vi "ModeMgr.Setup Utility.vi"() -> ()   [LabVIEW 2018]
uses:
  ModeMgr.Mode Settings.ctl
  ModeMgr.ModeConfig.ctl
  ModeMgr.Mode Settings_Config View.ctl
panel:
  in  "Delete Mode":bool
  in  "Mode List":i32(listbox)
  out "Option Descriptions":cluster{"Option":string, "Desc":string}[](array[cluster])=[{"Option"="Can Access Station Module", "Desc"="Level 0 = the button and menu item to open the station control module is not available.  Level 1 (or higher) = the station module can be opened."}, {"Option"="Can Clear Errors", "Desc"="Level 0 = the button to clear errors is disabled.  Level 1 (or higher) = the button to clear errors is enabled."}, {"Option"="Can Clear Warnings", "Desc"="Level 0 = the button to clear warnings is disabled.  Level 1 (or higher) = the button to clear warnings is enabled."}, {"Option"="Can Edit EQ List", "Desc"="Level 0 = the Equipment list can not be edited.  Level 1 (or higher) = the Equipment list can be edited."}, {"Option"="Can Edit Options", "Desc"="Level 0 = the controls for options (on tab page Config - Options) is disabled.  Level 1 (or higher) = the controls for options (on tab page Config - Options) is enabled."}, {"Option"="Can Generate Reports", "Desc"="Level 0 = the controls to generate RTF or CSV reports are disabled.  Level 1 (or higher) = the controls to generate RTF or CSV reports are enabled."}, {"Option"="Can Select Sequence", "Desc"="Level 0 = the controls for selecting the test sequence is disabled.  The default sequence (configured) is the only available sequenct that can be run. Level 1 (or higher) = the sequence selector control is enabled."}, {"Option"="Can View Config", "Desc"="Level 0 = the tab page for Config is hidden.  Level 1 (or higher) = the tab page for Config is visible and can eb selected."}, {"Option"="Disable Results", "Desc"="Level 0 = test results are reported for each test 9to Factory and to Data Warehouse).  Level 1 (or higher) = no results are reported."}, {"Option"="Disable Start with SN Entry", "Desc"="Level 0 = the control to auto start test when a SN is entered is set to ON and can not be changed.  Level 1 (or higher) = the control to auto start test when a SN is entered is set to OFF and can be changed by the operator."}, {"Option"="Display Result Data Details", "Desc"="\"Level 0 =  The operator can only view the summary page.  Level 1 (or higher) = the tabs of the result section will be displayed and the operator can select to view the Summary"}, {"Option"="Not Reset SN between Tests", "Desc"="Level 0 = the SN field is cleared between tests.  Level 1 (or higher) = the SN remains the same between tests."}, {"Option"="Not Validate Operator", "Desc"="Level 0 = the operator field can not be empty.  The Start button is disabled until the operator field is populated.  Level 1 (or higher) = the operator can be empty."}, {"Option"="Not Validate SN", "Desc"="Level 0 = the SN field can not be empty.  The Start button is disabled until the SN field is populated.  Level 1 (or higher) = the SN can be empty."}]
  in  "Add Mode":bool
  out "Options":string[](array[string])=["Option", "Display Result Data Details", "Not Reset SN between Tests", "Not Validate Operator", "Not Validate SN", "Disable Results", "Can Access Station Module", "Can Edit EQ List", "Can Clear Warnings", "Can Clear Errors", "Can View Config", "Can Edit Options", "Can Select Sequence", "Can Generate Reports", "Disable Start with SN Entry"]
  out "Options File":path
  out "Ver":string
  in  "Save":bool
  in  "Load":bool
  in  "Mode Config":cluster{"Default Mode":string, "Modes":T1[]}={"Default Mode"="Production", "Modes"=[{"Name"="Production", "Color"=3, "Options"=[{"Option"="Can Access Station Module", "Level"=0}, {"Option"="Can Clear Errors", "Level"=0}, {"Option"="Can Clear Warnings", "Level"=0}, {"Option"="Can Edit EQ List", "Level"=0}, {"Option"="Can Edit Options", "Level"=0}, {"Option"="Can Generate Reports", "Level"=0}, {"Option"="Can Select Sequence", "Level"=0}, {"Option"="Can View Config", "Level"=0}, {"Option"="Disable Results", "Level"=0}, {"Option"="Disable Start with SN Entry", "Level"=0}, {"Option"="Display Result Data Details", "Level"=0}, {"Option"="Not Reset SN between Tests", "Level"=0}, {"Option"="Not Validate Operator", "Level"=0}, {"Option"="Not Validate SN", "Level"=0}], "Password"=""}, {"Name"="Technician", "Color"=1, "Options"=[{"Option"="Can Access Station Module", "Level"=0}, {"Option"="Can Clear Errors", "Level"=1}, {"Option"="Can Clear Warnings", "Level"=1}, {"Option"="Can Edit EQ List", "Level"=0}, {"Option"="Can Edit Options", "Level"=0}, {"Option"="Can Generate Reports", "Level"=1}, {"Option"="Can Select Sequence", "Level"=1}, {"Option"="Can View Config", "Level"=0}, {"Option"="Disable Results", "Level"=0}, {"Option"="Disable Start with SN Entry", "Level"=1}, {"Option"="Display Result Data Details", "Level"=1}, {"Option"="Not Reset SN between Tests", "Level"=1}, {"Option"="Not Validate Operator", "Level"=1}, {"Option"="Not Validate SN", "Level"=0}], "Password"=""}, {"Name"="Gage R&R", "Color"=6, "Options"=[{"Option"="Can Access Station Module", "Level"=0}, {"Option"="Can Clear Errors", "Level"=0}, {"Option"="Can Clear Warnings", "Level"=0}, {"Option"="Can Edit EQ List", "Level"=0}, {"Option"="Can Edit Options", "Level"=0}, {"Option"="Can Generate Reports", "Level"=0}, {"Option"="Can Select Sequence", "Level"=0}, {"Option"="Can View Config", "Level"=0}, {"Option"="Disable Results", "Level"=0}, {"Option"="Disable Start with SN Entry", "Level"=0}, {"Option"="Display Result Data Details", "Level"=0}, {"Option"="Not Reset SN between Tests", "Level"=0}, {"Option"="Not Validate Operator", "Level"=0}, {"Option"="Not Validate SN", "Level"=0}], "Password"=""}, {"Name"="Engineering", "Color"=4, "Options"=[{"Option"="Can Access Station Module", "Level"=1}, {"Option"="Can Clear Errors", "Level"=1}, {"Option"="Can Clear Warnings", "Level"=1}, {"Option"="Can Edit EQ List", "Level"=1}, {"Option"="Can Edit Options", "Level"=1}, {"Option"="Can Generate Reports", "Level"=1}, {"Option"="Can Select Sequence", "Level"=1}, {"Option"="Can View Config", "Level"=1}, {"Option"="Disable Results", "Level"=1}, {"Option"="Disable Start with SN Entry", "Level"=1}, {"Option"="Display Result Data Details", "Level"=1}, {"Option"="Not Reset SN between Tests", "Level"=1}, {"Option"="Not Validate Operator", "Level"=1}, {"Option"="Not Validate SN", "Level"=1}], "Password"=""}]} {"Modes"."Color" items=["Red", "Yellow", "Orange", "Green", "SkyBlue", "Blue", "Purple", "Pink", "Grey"]}
  # "MTE Mode Setup Utility"
  # "Option                                                                                             Description"
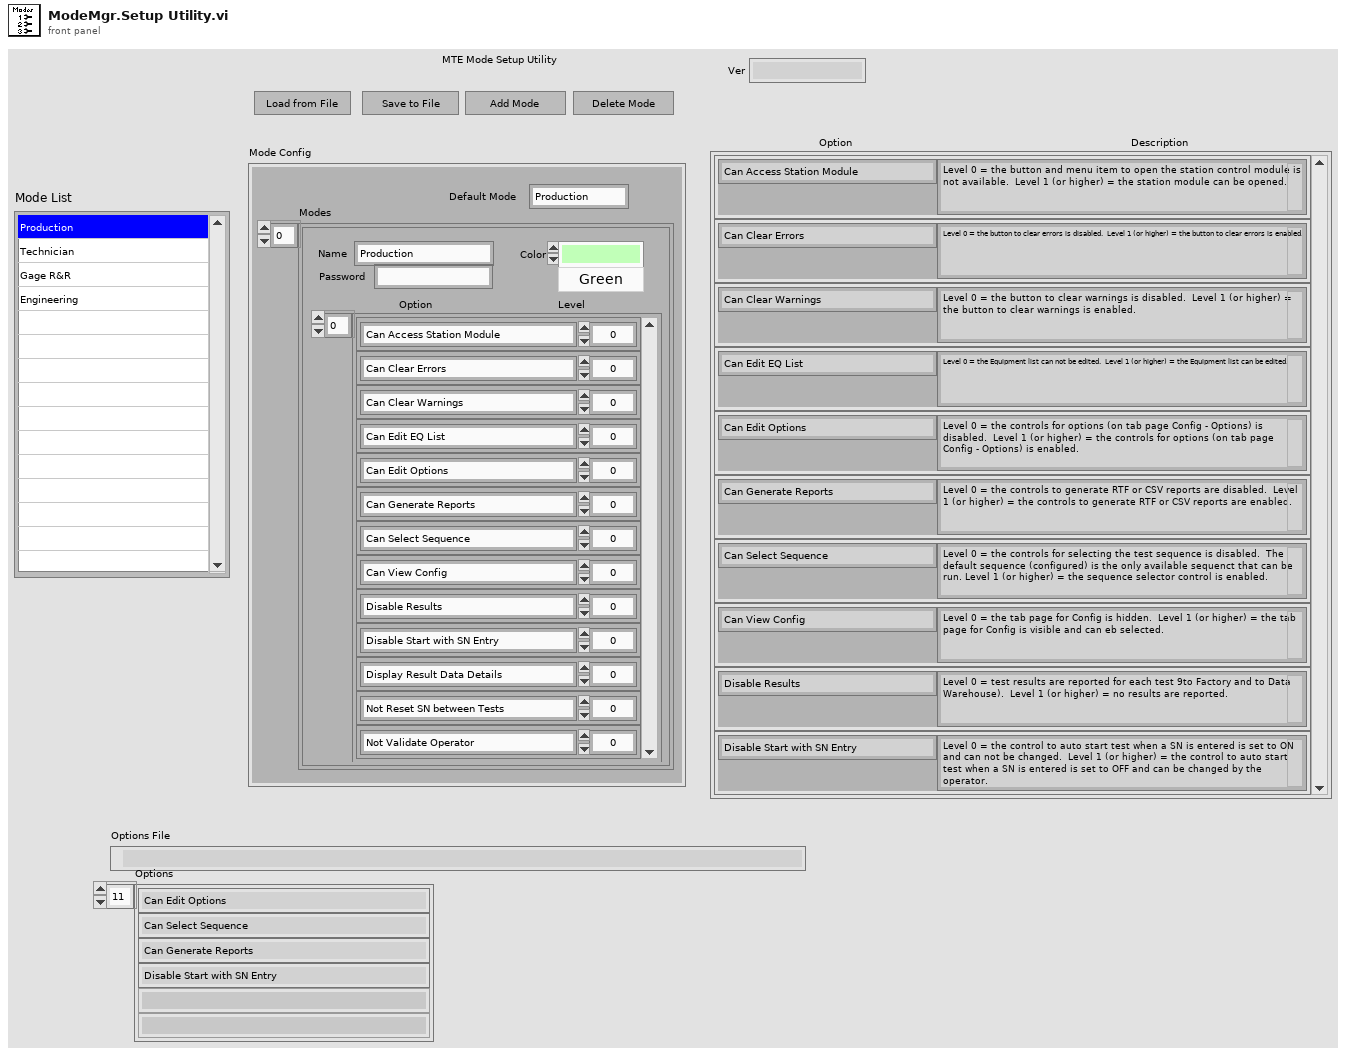
[diagram p1: front panel]
types:
  T1 = typedef "ModeMgr.Mode Settings_Config View.ctl" = cluster{"Name":string, "Color":u16, "Options":T2[], "Password":string}
  T2 = typedef "ModeMgr.Mode Settings.ctl" = cluster{"Option":string, "Level":i32}
  T3 = enum32{"invalid app kind", "Development System", "Run Time System", "Student Edition", "Embedded LabVIEW", "Evaluation", "Custom"}
  T4 = typedef "ModeMgr.ModeConfig.ctl" = cluster{"Name":string, "Color":string, "Settings":T2[], "Password":string}
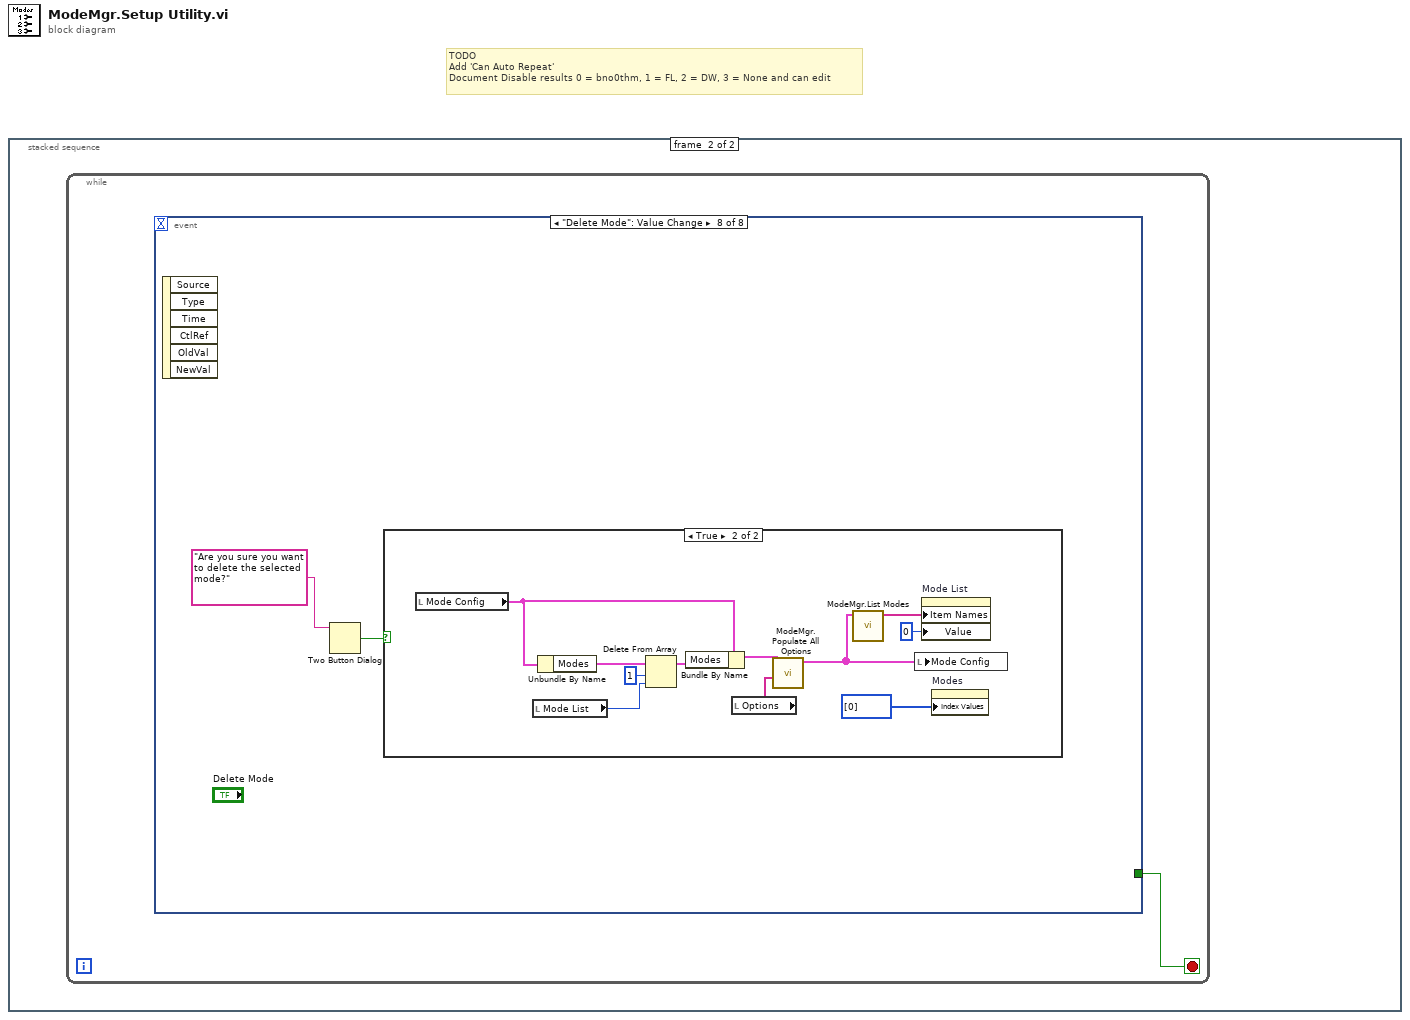
[diagram p0: block diagram]
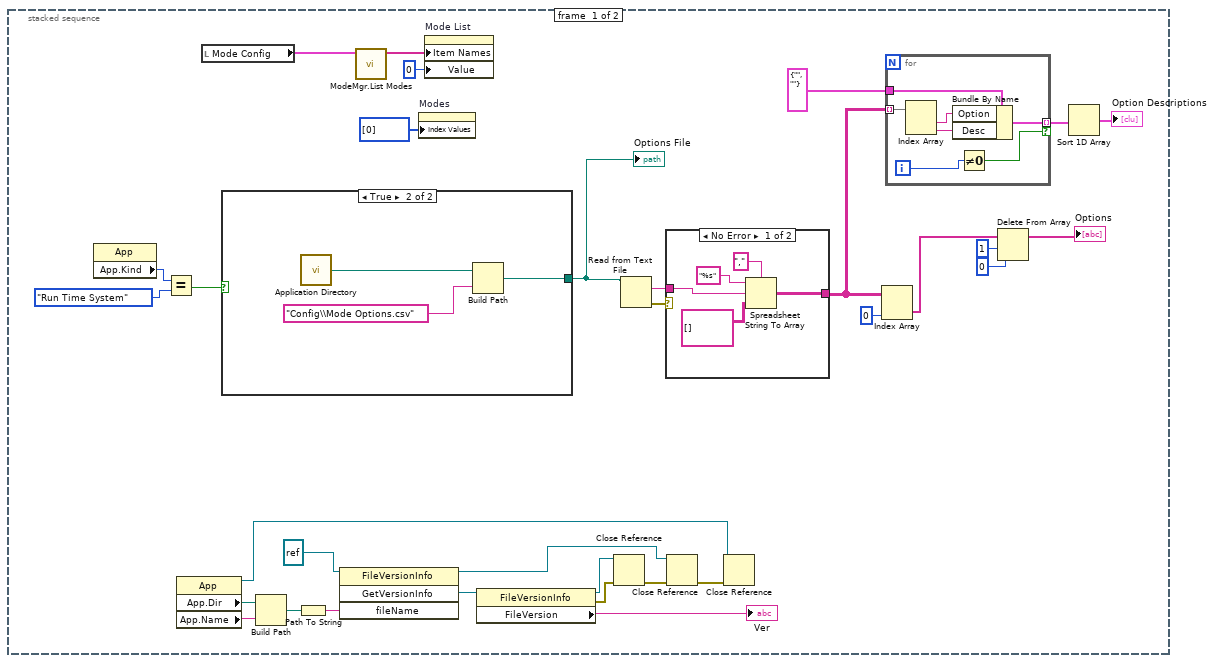
[diagram p2: hidden frame]
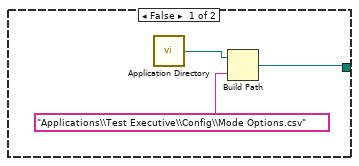
[diagram p4: hidden frame]
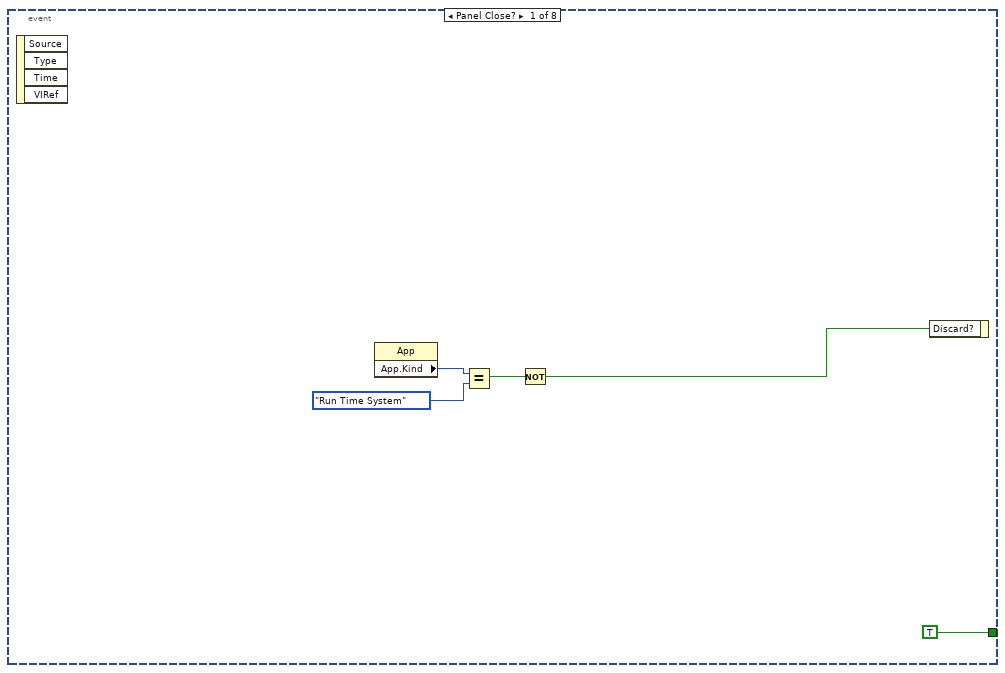
[diagram p5: hidden frame]
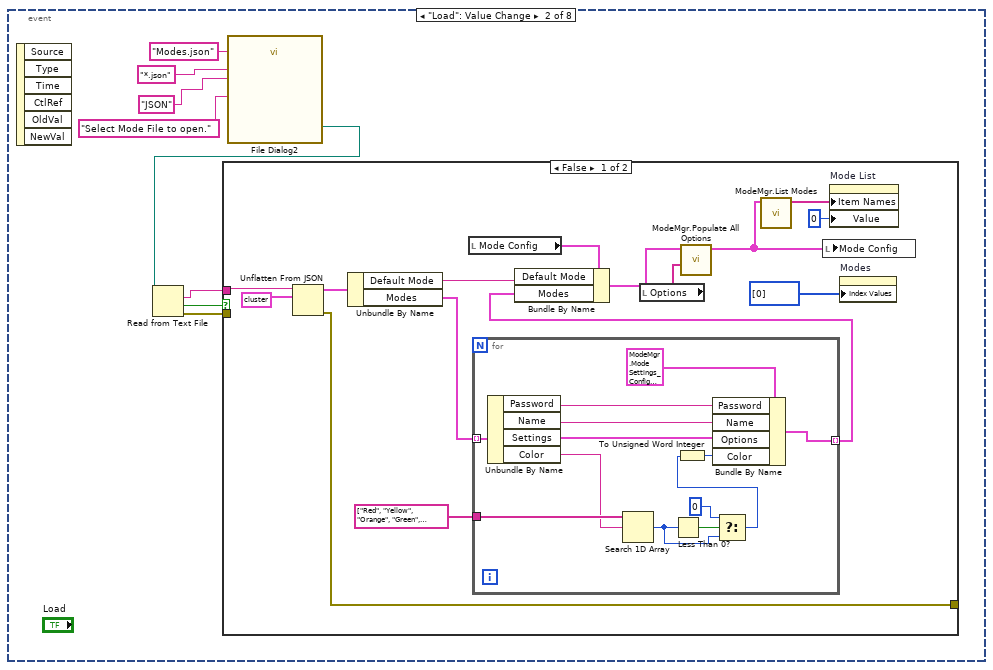
[diagram p6: hidden frame]
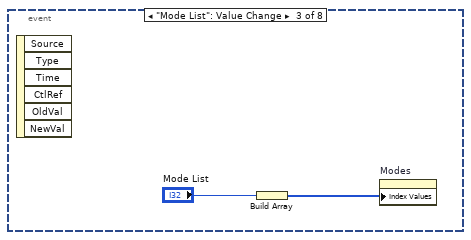
[diagram p8: hidden frame]
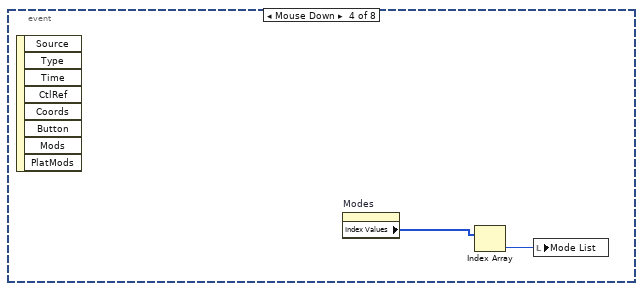
[diagram p9: hidden frame]
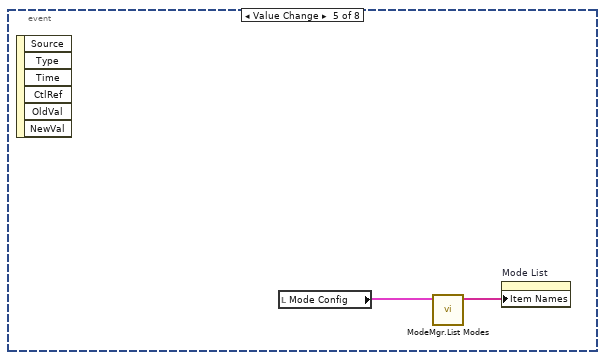
[diagram p10: hidden frame]
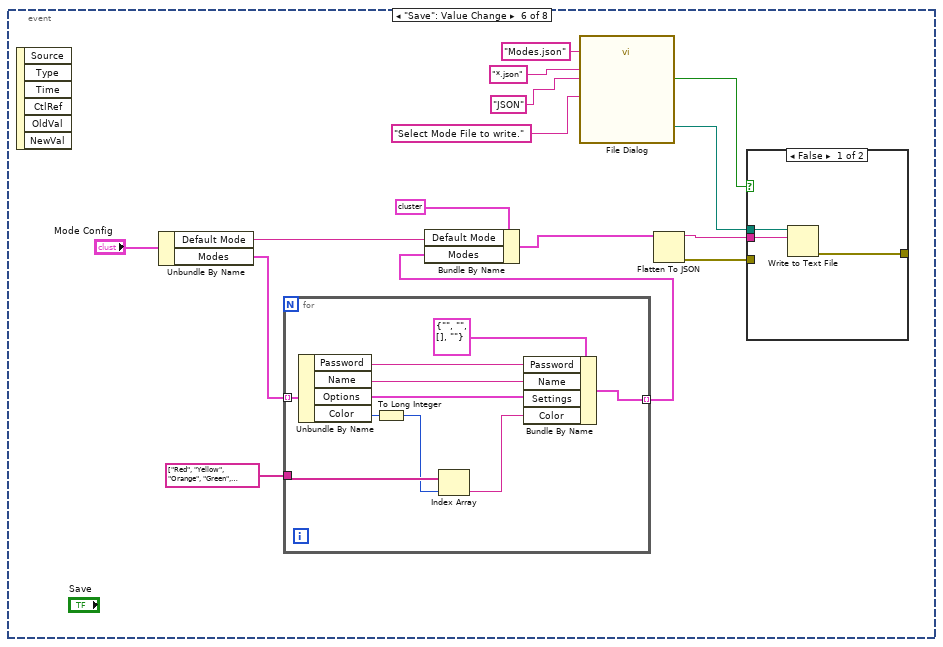
[diagram p11: hidden frame]
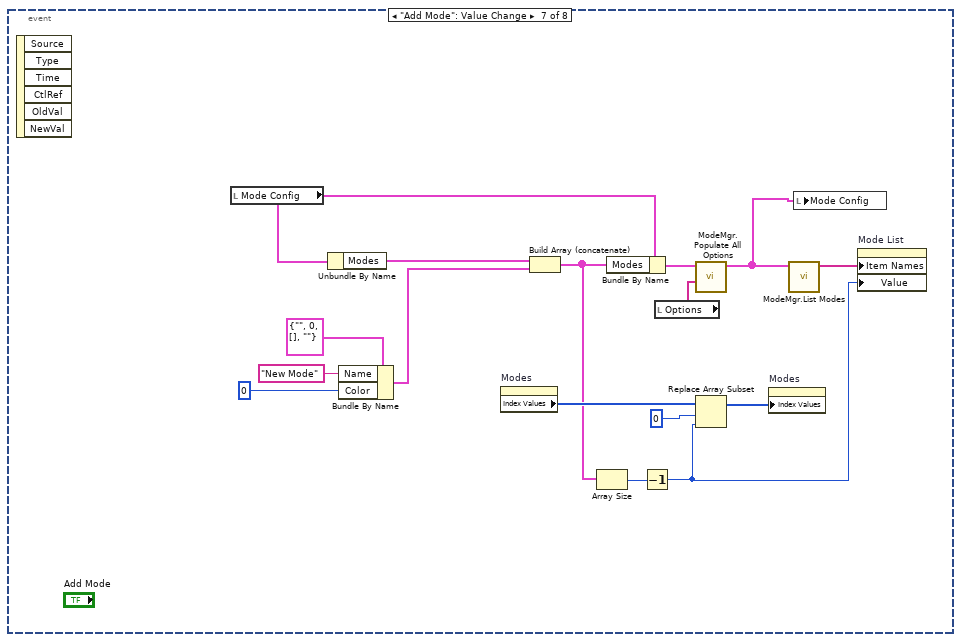
[diagram p13: hidden frame]
diagram:
  # "TODO\nAdd 'Can Auto Repeat'\nDocument Disable results 0 = bno0thm, 1 = FL, 2 = DW, 3 = None and can edit"
  n1 = stacked-sequence {
    frame #0 {
      n2 = property class="App"() -> ("App.Kind"=w32:T3)  [unwired: 2 in, 2 out]
      n3 = Equal?(x=w32, y=T3."Run Time System" ("Application:Kind")) -> (x = y?=w17:bool)
      n4 = property class="App"() -> (reference out=w29:refnum<vi>, "App.Dir"=w25:path, "App.Name"=w26:string)  [unwired: 2 in, 1 out]
      n5 = local read "Mode Config"() -> (w9:cluster{"Default Mode":string, "Modes":T1[]})
      n6 = case shown="True" w17 {
        tunnel: [w45 w48] -> w16
        frame False {
          n7 = call <vilib>:"Application Directory.vi"() -> ("Application Directory"=w46:path)
          n8 = Build Path(base path=w46, name or relative path="Applications\\Test Executive\\Config\\Mode Options.csv") -> (appended path=w45:path)
        }
        frame True {
          n9 = call <vilib>:"Application Directory.vi"() -> ("Application Directory"=w50:path)
          n10 = Build Path(base path=w50, name or relative path="Config\\Mode Options.csv") -> (appended path=w48:path)
        }
      }
      "Options File" <- w16
      n11 = Build Path(base path=w25, name or relative path=w26) -> (appended path=w27:path)
      n12 = Path To String(path=w27) -> (string=w20:string)
      n13 = invoke class="FileVersionInfo" method="GetVersionInfo"(reference=refnum<k24> refnum, "fileName"=w20) -> (reference out=w24:refnum<k24>, "GetVersionInfo"=w19:refnum<k24>)  [unwired: 2 in, 2 out]
      n14 = call "ModeMgr.List Modes.vi"("Modes"=w9) -> ("Names"=w8:string[])  [unwired: 10 in]
      n15 = property on="Modes" class="Arr (strict)"("Index Values"=u32[] [0]) -> ()  [unwired: 2 in, 2 out]
      n16 = property on="Mode List" class="LstBox (strict)"("Item Names"=w8, "Value"=0 ("Modes")) -> ()  [unwired: 2 in, 2 out]
      n17 = property class="FileVersionInfo"(reference=w19) -> (reference out=w21:refnum<k24>, error out=w22:errorcluster, "FileVersion"=→"Ver":string)  [unwired: 1 in]
      n18 = Close Reference(reference=w21, error in (no error)=w22) -> (error out=w23:errorcluster)
      n19 = Read from Text File(file (use dialog)=w16) -> (text=w14:string, error out=w15:errorcluster)  [unwired: 3 in, 2 out]
      n20 = case shown="No Error" w15 {
        tunnel: w14 -> [w43 _]
        tunnel: [w40 _] -> w1
        frame No Error {
          n21 = Spreadsheet String To Array(delimiter (Tab)=",", format string="%s", spreadsheet string=w43, array type (2D Dbl)=string[][] []) -> (array=w40:string[][])
        }
        frame Error {
        }
      }
      n22 = Close Reference(reference=w24, error in (no error)=w23) -> (error out=w28:errorcluster)
      n23 = Close Reference(reference=w29, error in (no error)=w28) -> ()  [unwired: 1 out]
      n24 = Index Array(array=w1, index (col)=0 ("disabled index (col)")) -> (element=w5:string[])  [unwired: 1 in]
      n25 = for {
        tunnel: w1 -> [w38] mode=indexing
        tunnel: cluster{"Option":string, "Desc":string} {"Option"="", "Desc"=""} ("Cluster") -> [w39]
        tunnel: [w37] -> w11 mode=indexing if=w33
        i -> [w34]
        n26 = Index Array(array=w38) -> (element #1=w36:string, element #2=w35:string)  [unwired: 2 in]
        n27 = Bundle By Name(cluster=w39, "Option"=w36, "Desc"=w35) -> (w37:cluster{"Option":string, "Desc":string})
        n28 = Not Equal To 0?(x=w34) -> (x != 0?=w33:bool)
      }
      n29 = Delete From Array(array=w5, length=1, index=0) -> (array with subset deleted=→"Options":string[])  [unwired: 1 out]
      n30 = Sort 1D Array(array=w11) -> (sorted array=→"Option Descriptions":cluster{"Option":string, "Desc":string}[])
    }
    frame #1 {
      n31 = while {
        stop <- w51 stop-if-true
        n32 = event shown="[7] \"Delete Mode\": Value Change" {
          selector: _ -> [_ _ _ _ _ _ _ _]
          dyn-events: _ -> [_ _ _ _ _ _ _ _]
          timeout: _ -> [_ _ _ _ _ _ _ _]
          tunnel: [TRUE _ _ _ _ _ _ _] -> w51
          event Panel Close? {
            n33 = event-data() -> ()  [unwired: 1 in, 4 out]
            n34 = property class="App"() -> ("App.Kind"=w55:T3)  [unwired: 2 in, 2 out]
            n35 = Equal?(x=w55, y=T3."Run Time System" ("Application:Kind")) -> (x = y?=w53:bool)
            n36 = Not(x=w53) -> (.not. x?=w52:bool)
            n37 = event-data("Discard?"=w52) -> ()  [unwired: 1 in, 1 out]
          }
          event "Load": Value Change {
            n38 = event-data() -> ()  [unwired: 1 in, 6 out]
            n39 = call "File Dialog2"("prompt"="Select Mode File to open." ("prompt (Choose or enter file path)"), "default name"="Modes.json", "pattern (all files)"="*.json", "pattern label"="JSON" ("pattern (all files)")) -> ("selected path"=w57:path)  [unwired: 8 in, 3 out]
            n40 = Read from Text File(file (use dialog)=w57) -> (text=w63:string, cancelled=w64:bool, error out=w62:errorcluster)  [unwired: 3 in, 1 out]
            n41 = case shown="False" w64 {
              tunnel: w63 -> [w79 _]
              tunnel: [w72 _] -> _
              tunnel: w62 -> [_ _]
              frame False {
                n42 = Unflatten From JSON(JSON string=w79, type and defaults=cluster{"Default Mode":string, "Modes":T4[]} {"Default Mode"="Production", "Modes"=[{"Name"="Production", "Color"="Green", "Settings"=[{"Option"="PreTest_Validate_SN", "Level"=1}, {"Option"="PostTest_ReportResult", "Level"=1}, {"Option"="OptTo_NotSaveResults", "Level"=0}, {"Option"="OptTo_NotStopOnFail", "Level"=0}, {"Option"="OptTo_SetConfig", "Level"=0}, {"Option"="OptTo_UpdateEquipmentList", "Level"=0}, {"Option"="OptTo_AccessManualStaControl", "Level"=0}], "Password"=""}, {"Name"="Technician", "Color"="Yellow", "Settings"=[{"Option"="PreTest_Validate_SN", "Level"=0}, {"Option"="PostTest_ReportResult", "Level"=0}, {"Option"="OptTo_NotSaveResults", "Level"=1}, {"Option"="OptTo_NotStopOnFail", "Level"=1}, {"Option"="OptTo_SetConfig", "Level"=0}, {"Option"="OptTo_UpdateEquipmentList", "Level"=0}, {"Option"="OptTo_AccessManualStaControl", "Level"=0}], "Password"=""}, {"Name"="Engineering", "Color"="SkyBlue", "Settings"=[{"Option"="PreTest_Validate_SN", "Level"=0}, {"Option"="PostTest_ReportResult", "Level"=0}, {"Option"="OptTo_NotSaveResults", "Level"=1}, {"Option"="OptTo_NotStopOnFail", "Level"=1}, {"Option"="OptTo_SetConfig", "Level"=1}, {"Option"="OptTo_UpdateEquipmentList", "Level"=1}, {"Option"="OptTo_AccessManualStaControl", "Level"=1}], "Password"=""}, {"Name"="Production", "Color"="Green", "Settings"=[], "Password"=""}, {"Name"="Technician", "Color"="Yellow", "Settings"=[], "Password"=""}, {"Name"="Engineering", "Color"="Blue", "Settings"=[], "Password"=""}]} ("Mode Config")) -> (value=w77:cluster{"Default Mode":string, "Modes":T4[]}, error out=w72:errorcluster)  [unwired: 5 in]
                n43 = Unbundle By Name(w77) -> ("Default Mode"=w75:string, "Modes"=w74:T4[])
                n44 = local read "Mode Config"() -> (w76:cluster{"Default Mode":string, "Modes":T1[]})
                n45 = for {
                  tunnel: w74 -> [w92] mode=indexing
                  tunnel: string[] ["Red", "Yellow", "Orange", "Green", "SkyBlue", "Blue", "Purple", "Pink", "Grey"] ("Names") -> [w89]
                  tunnel: [w82] -> w71 mode=indexing
                  n46 = Unbundle By Name(w92) -> ("Password"=w80:string, "Name"=w91:string, "Settings"=w90:T2[], "Color"=w88:string)
                  n47 = Search 1D Array(1D array=w89, element=w88) -> (index of element=w86:i32)  [unwired: 1 in]
                  n48 = Less Than 0?(x=w86) -> (x < 0?=w87:bool)
                  n49 = Select(t=0, s=w87, f=w86) -> (s? t:f=w84:i32)
                  n50 = To Unsigned Word Integer(number=w84) -> (unsigned 16bit integer=w83:u16)
                  n51 = Bundle By Name(cluster=T1 {"Name"="Production", "Color"=3, "Options"=[{"Option"="Can Access Station Module", "Level"=0}, {"Option"="Can Clear Errors", "Level"=0}, {"Option"="Can Clear Warnings", "Level"=0}, {"Option"="Can Edit EQ List", "Level"=0}, {"Option"="Can Edit Options", "Level"=0}, {"Option"="Can Generate Reports", "Level"=0}, {"Option"="Can Select Sequence", "Level"=0}, {"Option"="Can View Config", "Level"=0}, {"Option"="Disable Results", "Level"=0}, {"Option"="Disable Start with SN Entry", "Level"=0}, {"Option"="Display Result Data Details", "Level"=0}, {"Option"="Not Reset SN between Tests", "Level"=0}, {"Option"="Not Validate Operator", "Level"=0}, {"Option"="Not Validate SN", "Level"=0}], "Password"=""} ("Config"), "Password"=w80, "Name"=w91, "Options"=w90, "Color"=w83) -> (w82:T1)
                }
                n52 = Bundle By Name(cluster=w76, "Default Mode"=w75, "Modes"=w71) -> (w70:cluster{"Default Mode":string, "Modes":T1[]})
                n53 = local read "Options"() -> (w69:string[])
                n54 = call "ModeMgr.Populate All Options.vi"("Options"=w69, "Modes"=w70) -> ("Modes Out"=w65:T1[])  [unwired: 9 in]
                n55 = call "ModeMgr.List Modes.vi"("Modes"=w65) -> ("Names"=w67:string[])  [unwired: 10 in]
                n56 = local write "Mode Config"(w65) -> ()
                n57 = property on="Mode List" class="LstBox (strict)"("Item Names"=w67, "Value"=0 ("Modes")) -> ()  [unwired: 2 in, 2 out]
                n58 = property on="Modes" class="Arr (strict)"("Index Values"=u32[] [0]) -> ()  [unwired: 2 in, 2 out]
              }
              frame True {
                # "Do nothing.  Canceled"
              }
            }
          }
          event "Mode List": Value Change {
            n59 = event-data() -> ()  [unwired: 1 in, 6 out]
            n60 = Build Array("Mode List") -> (w93:i32[])
            n61 = property on="Modes" class="Arr (strict)"("Index Values"=w93) -> ()  [unwired: 2 in, 2 out]
          }
          event "Mode Config.Modes": Mouse Down {
            n62 = event-data() -> ()  [unwired: 1 in, 8 out]
            n63 = property on="Modes" class="Arr (strict)"() -> ("Index Values"=w95:u32[])  [unwired: 2 in, 2 out]
            n64 = Index Array(array=w95) -> (element=w96:u32)  [unwired: 1 in]
            n65 = local write "Mode List"(w96) -> ()
          }
          event "Mode Config.Modes": Value Change {
            n66 = event-data() -> ()  [unwired: 1 in, 6 out]
            n67 = local read "Mode Config"() -> (w98:cluster{"Default Mode":string, "Modes":T1[]})
            n68 = call "ModeMgr.List Modes.vi"("Modes"=w98) -> ("Names"=w97:string[])  [unwired: 10 in]
            n69 = property on="Mode List" class="LstBox (strict)"("Item Names"=w97) -> ()  [unwired: 2 in, 2 out]
          }
          event "Save": Value Change {
            n70 = event-data() -> ()  [unwired: 1 in, 6 out]
            n71 = Unbundle By Name("Mode Config") -> ("Default Mode"=w113:string, "Modes"=w112:T1[])
            n72 = for {
              tunnel: w112 -> [w126] mode=indexing
              tunnel: string[] ["Red", "Yellow", "Orange", "Green", "SkyBlue", "Blue", "Purple", "Pink", "Grey"] ("Names") -> [w121]
              tunnel: [w123] -> w110 mode=indexing
              n73 = Unbundle By Name(w126) -> ("Password"=w117:string, "Name"=w125:string, "Options"=w124:T2[], "Color"=w120:u16)
              n74 = To Long Integer(number=w120) -> (32bit integer=w119:i32)
              n75 = Index Array(array=w121, index=w119) -> (element=w118:string)
              n76 = Bundle By Name(cluster=T4 {"Name"="", "Color"="", "Settings"=[], "Password"=""} ("Config"), "Password"=w117, "Name"=w125, "Settings"=w124, "Color"=w118) -> (w123:T4)
            }
            n77 = Bundle By Name(cluster=cluster{"Default Mode":string, "Modes":T4[]} {"Default Mode"="Production", "Modes"=[{"Name"="Production", "Color"="Green", "Settings"=[{"Option"="PreTest_Validate_SN", "Level"=1}, {"Option"="PostTest_ReportResult", "Level"=1}, {"Option"="OptTo_NotSaveResults", "Level"=0}, {"Option"="OptTo_NotStopOnFail", "Level"=0}, {"Option"="OptTo_SetConfig", "Level"=0}, {"Option"="OptTo_UpdateEquipmentList", "Level"=0}, {"Option"="OptTo_AccessManualStaControl", "Level"=0}], "Password"=""}, {"Name"="Technician", "Color"="Yellow", "Settings"=[{"Option"="PreTest_Validate_SN", "Level"=0}, {"Option"="PostTest_ReportResult", "Level"=0}, {"Option"="OptTo_NotSaveResults", "Level"=1}, {"Option"="OptTo_NotStopOnFail", "Level"=1}, {"Option"="OptTo_SetConfig", "Level"=0}, {"Option"="OptTo_UpdateEquipmentList", "Level"=0}, {"Option"="OptTo_AccessManualStaControl", "Level"=0}], "Password"=""}, {"Name"="Engineering", "Color"="SkyBlue", "Settings"=[{"Option"="PreTest_Validate_SN", "Level"=0}, {"Option"="PostTest_ReportResult", "Level"=0}, {"Option"="OptTo_NotSaveResults", "Level"=1}, {"Option"="OptTo_NotStopOnFail", "Level"=1}, {"Option"="OptTo_SetConfig", "Level"=1}, {"Option"="OptTo_UpdateEquipmentList", "Level"=1}, {"Option"="OptTo_AccessManualStaControl", "Level"=1}], "Password"=""}, {"Name"="Production", "Color"="Green", "Settings"=[], "Password"=""}, {"Name"="Technician", "Color"="Yellow", "Settings"=[], "Password"=""}, {"Name"="Engineering", "Color"="Blue", "Settings"=[], "Password"=""}]} ("Mode Config"), "Default Mode"=w113, "Modes"=w110) -> (w107:cluster{"Default Mode":string, "Modes":T4[]})
            n78 = call "File Dialog"("prompt"="Select Mode File to write." ("prompt (Choose or enter file path)"), "default name"="Modes.json", "pattern (all files)"="*.json", "pattern label"="JSON" ("pattern (all files)")) -> ("selected path"=w102:path, "cancelled"=w101:bool)  [unwired: 8 in, 2 out]
            n79 = Flatten To JSON(anything=w107) -> (JSON string=w106:string, 11:w100:errorcluster)  [unwired: 2 in]
            n80 = case shown="False" w101 {
              tunnel: w106 -> [w116 _]
              tunnel: w102 -> [w115 _]
              tunnel: [w114 _] -> _
              tunnel: w100 -> [_ _]
              frame False {
                n81 = Write to Text File(file (use dialog)=w115, text=w116) -> (error out=w114:errorcluster)  [unwired: 2 in, 2 out]
              }
              frame True {
              }
            }
          }
          event "Add Mode": Value Change {
            n82 = event-data() -> ()  [unwired: 1 in, 6 out]
            n83 = local read "Mode Config"() -> (w141:cluster{"Default Mode":string, "Modes":T1[]})
            n84 = Unbundle By Name(w141) -> ("Modes"=w142:T1[])
            n85 = Bundle By Name(cluster=T1 {"Name"="", "Color"=0, "Options"=[], "Password"=""} ("Config"), "Name"="New Mode", "Color"=u16 0) -> (w135:T1)
            n86 = property on="Modes" class="Arr (strict)"() -> ("Index Values"=w140:u32[])  [unwired: 2 in, 2 out]
            n87 = Build Array (concatenate)(w142, w135) -> (w137:T1[])
            n88 = Array Size(array=w137) -> (size(s)=w129:i32)
            n89 = Bundle By Name(cluster=w141, "Modes"=w137) -> (w130:cluster{"Default Mode":string, "Modes":T1[]})
            n90 = Decrement(x=w129) -> (x-1=w128:i32)
            n91 = local read "Options"() -> (w132:string[])
            n92 = call "ModeMgr.Populate All Options.vi"("Options"=w132, "Modes"=w130) -> ("Modes Out"=w131:T1[])  [unwired: 9 in]
            n93 = Replace Array Subset(array=w140, new element=w128, index=0) -> (w139:u32[])
            n94 = property on="Modes" class="Arr (strict)"("Index Values"=w139) -> ()  [unwired: 2 in, 2 out]
            n95 = call "ModeMgr.List Modes.vi"("Modes"=w131) -> ("Names"=w136:string[])  [unwired: 10 in]
            n96 = local write "Mode Config"(w131) -> ()
            n97 = property on="Mode List" class="LstBox (strict)"("Item Names"=w136, "Value"=w128) -> ()  [unwired: 2 in, 2 out]
          }
          event "Delete Mode": Value Change {
            n98 = event-data() -> ()  [unwired: 1 in, 6 out]
            n99 = Two Button Dialog(message="Are you sure you want to delete the selected mode?") -> (T button?=w143:bool)  [unwired: 2 in]
            n100 = case shown="True" w143 {
              frame False {
              }
              frame True {
                n101 = local read "Mode Config"() -> (w155:cluster{"Default Mode":string, "Modes":T1[]})
                n102 = local read "Mode List"() -> (w151:i32)
                n103 = Unbundle By Name(w155) -> ("Modes"=w154:T1[])
                n104 = Delete From Array(array=w154, length=1, index=w151) -> (array with subset deleted=w153:T1[])  [unwired: 1 out]
                n105 = Bundle By Name(cluster=w155, "Modes"=w153) -> (w145:cluster{"Default Mode":string, "Modes":T1[]})
                n106 = local read "Options"() -> (w150:string[])
                n107 = call "ModeMgr.Populate All Options.vi"("Options"=w150, "Modes"=w145) -> ("Modes Out"=w146:T1[])  [unwired: 9 in]
                n108 = call "ModeMgr.List Modes.vi"("Modes"=w146) -> ("Names"=w148:string[])  [unwired: 10 in]
                n109 = local write "Mode Config"(w146) -> ()
                n110 = property on="Mode List" class="LstBox (strict)"("Item Names"=w148, "Value"=0 ("Modes")) -> ()  [unwired: 2 in, 2 out]
                n111 = property on="Modes" class="Arr (strict)"("Index Values"=u32[] [0]) -> ()  [unwired: 2 in, 2 out]
              }
            }
          }
        }
      }
    }
  }
